vi "Set State_Measure SMU_HOLD.vi"(4 "Hold Time (s)":dbl=1.0 caption="Delay Time (s)", 6 "SMU Settings":T2={"Level"=0.01, "Level Range"=0.1, "Limit"=1.0, "Limit Range"=6.0, "Sense"=1009} {"Sense" items=["Local"=1008, "Remote"=1009]}, 7 "script name":string, 8 "error in (no error)":errorcluster, 9 "Published Data Id":string, 10 "Pins":string[](array[string])=["VDD"], 11 "Semiconductor Module Context":T3) -> (0 "error Out":errorcluster)   [LabVIEW 2013]
uses:
  <vilib>/NI_TestStand_SemiconductorModule/NI_TestStand_Semiconductor_Module.lvlibp/PinMap/General/SemiconductorModuleContext.ctl
  <instrlib>/niDCPower/nidcpower.llb/niDCPower Sense.ctl
  <instrlib>/niHSDIO/niHSDIO.llb/niHSDIO_ctl Trigger Script - trigID Values (Ring).ctl
  <vilib>/NI_TestStand_SemiconductorModule/NI_TestStand_Semiconductor_Module.lvlibp
panel:
  out "R Array":dbl[][](array[numeric]) format="%#_6p"
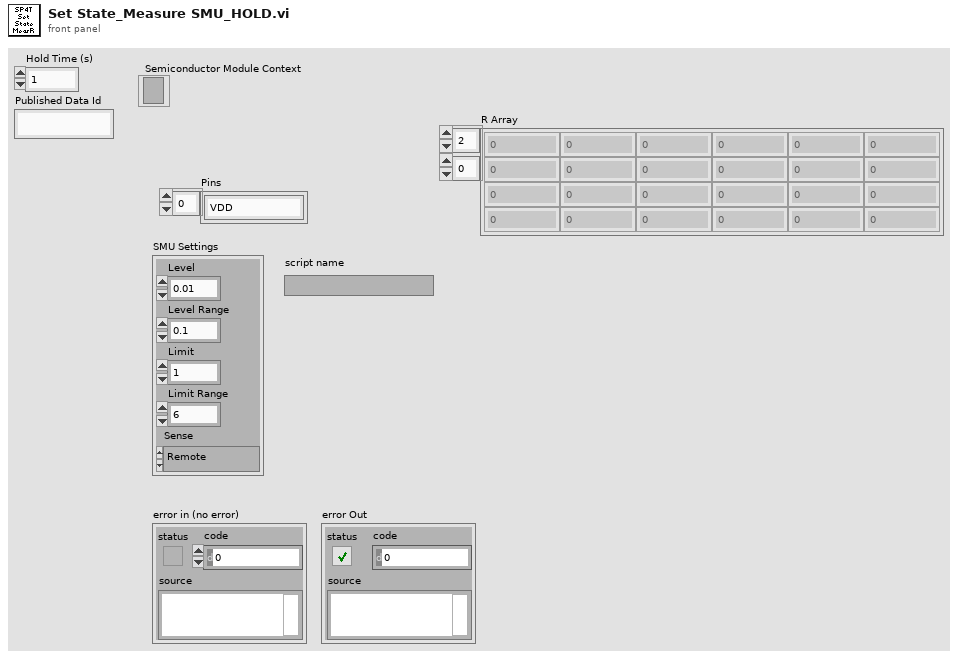
[diagram p1: front panel]
types:
  T1 = typedef "niDCPower Sense.ctl" = i32
  T2 = cluster{"Level":dbl, "Level Range":dbl, "Limit":dbl, "Limit Range":dbl, "Sense":T1}
  T3 = typedef "NI_TestStand_Semiconductor_Module.lvlibp/SemiconductorModuleContext.ctl" = refnum<k7>
  T4 = typedef "niHSDIO_ctl Trigger Script - trigID Values (Ring).ctl" = string
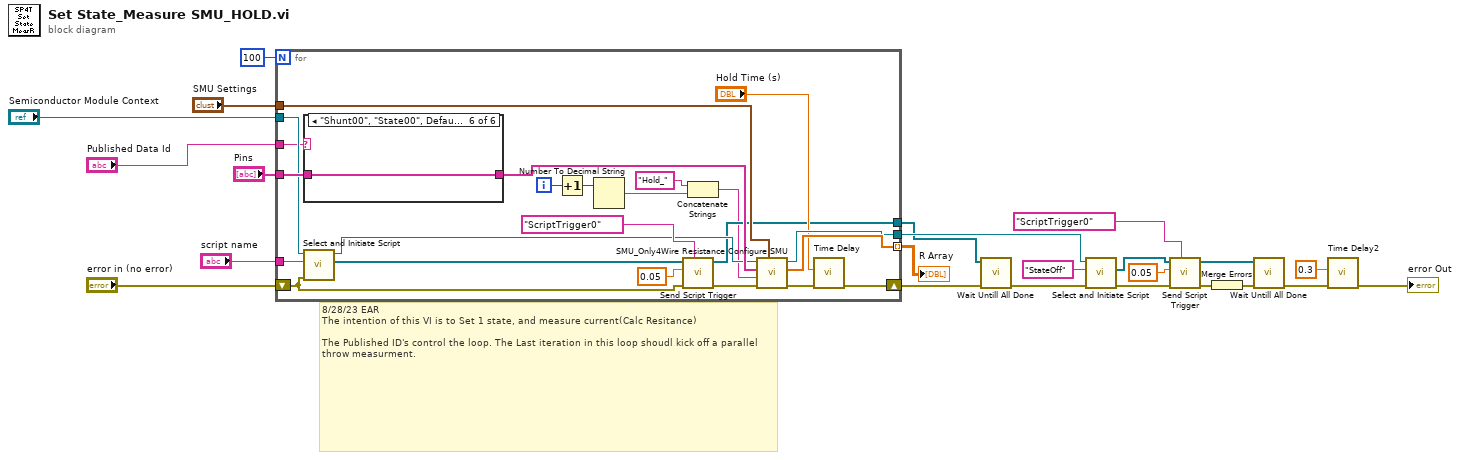
[diagram p0: block diagram]
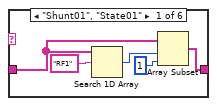
[diagram p2: hidden frame]
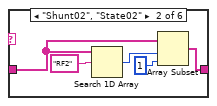
[diagram p3: hidden frame]
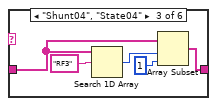
[diagram p4: hidden frame]
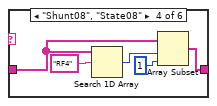
[diagram p5: hidden frame]
diagram:
  # "8/28/23 EAR\nThe intention of this VI is to Set 1 state, and measure current(Calc Resitance)\n\nThe Published ID's control the loop. The Last iteration in this loop shoudl kick off a parallel throw measurment."
  n1 = for {
    N: 100 -> [_]
    tunnel: "SMU Settings" -> [w46]
    tunnel: "Pins" -> [w42]
    tunnel: [w43] -> w21 mode=indexing
    shift-right: [w32] -> w6
    shift-left: "error in (no error)" -> [w35]
    tunnel: "Semiconductor Module Context" -> [w37]
    tunnel: "script name" -> [w36]
    tunnel: [w34] -> w11
    tunnel: "Published Data Id" -> [w30]
    tunnel: [w29] -> w4
    i -> [w25]
    n2 = case shown="\"Shunt00\", \"State00\", Default" w30 {
      tunnel: w42 -> [w50 w53 w60 w62 w67 w68]
      tunnel: [w49 w52 w59 w63 w67 w68] -> w41
      frame "Shunt01", "State01" {
        n3 = Search 1D Array(1D array=w50, element="RF1") -> (index of element=w48:i32)  [unwired: 1 in]
        n4 = Array Subset(array=w50, index=w48, length=1) -> (w49:string[])
      }
      frame "Shunt02", "State02" {
        n5 = Search 1D Array(1D array=w53, element="RF2") -> (index of element=w55:i32)  [unwired: 1 in]
        n6 = Array Subset(array=w53, index=w55, length=1) -> (w52:string[])
      }
      frame "Shunt04", "State04" {
        n7 = Search 1D Array(1D array=w60, element="RF3") -> (index of element=w58:i32)  [unwired: 1 in]
        n8 = Array Subset(array=w60, index=w58, length=1) -> (w59:string[])
      }
      frame "Shunt08", "State08" {
        n9 = Search 1D Array(1D array=w62, element="RF4") -> (index of element=w65:i32)  [unwired: 1 in]
        n10 = Array Subset(array=w62, index=w65, length=1) -> (w63:string[])
      }
      frame "Shunt15", "State15" {
      }
      frame "Shunt00", "State00", Default {
      }
    }
    n11 = call "Select and Initiate Script.vi"("error in (no error)"=w35, "script name"=w36, "Semiconductor Module Context"=w37) -> ("HSDIO GEN Sessions Out"=w39:refnum<k15>[], "Semiconductor Module Context Out"=w38:T3)  [unwired: 6 in, 1 out]
    n12 = Increment(x=w25) -> (x+1=w24:i32)
    n13 = Number To Decimal String(number=w24) -> (decimal integer string=w27:string)  [unwired: 1 in]
    n14 = call "Send Script Trigger.vi"("trigger id (script trigger 0)"=T4 "ScriptTrigger0", "error in (no error)"=w35, "Delay Time (s)"=0.05, "HSDIO Sessions In"=w39) -> ("error out"=w44:errorcluster, "HSDIO Sessions Out"=w29:refnum<k15>[])  [unwired: 6 in]
    n15 = Concatenate Strings("Hold_" ("string"), w27) -> (w26:string)
    n16 = call "SMU_Only4Wire Resistance Configure SMU.vi"("SMU Settings"=w46, "error in (no error)"=w44, "Published Data Id"=w26, "Pins"=w41, "Semiconductor Module Context"=w38) -> ("error Out"=w33:errorcluster, "R Array"=w43:dbl[], "Semiconductor Module Context Out"=w34:T3)  [unwired: 4 in]
    n17 = call "Time Delay"("error in (no error)"=w33, "Delay Time (s)"="Hold Time (s)") -> ("error out"=w32:errorcluster)  [unwired: 9 in]
  }
  "R Array" <- w21
  n18 = call "Wait Untill All Done.vi"("error in (no error)"=w6, "HSDIO Sessions In"=w4) -> ("error out"=w5:errorcluster)  [unwired: 8 in, 1 out]
  n19 = call "Select and Initiate Script.vi"("error in (no error)"=w5, "script name"="StateOff", "Semiconductor Module Context"=w11) -> ("error out"=w12:errorcluster, "HSDIO GEN Sessions Out"=w9:refnum<k15>[])  [unwired: 6 in, 1 out]
  n20 = call "Send Script Trigger.vi"("trigger id (script trigger 0)"=T4 "ScriptTrigger0", "error in (no error)"=w12, "Delay Time (s)"=0.05, "HSDIO Sessions In"=w9) -> ("error out"=w18:errorcluster, "HSDIO Sessions Out"=w17:refnum<k15>[])  [unwired: 6 in]
  n21 = Merge Errors(w18) -> (w20:errorcluster)
  n22 = call "Wait Untill All Done.vi"("error in (no error)"=w20, "HSDIO Sessions In"=w17) -> ("error out"=w3:errorcluster)  [unwired: 8 in, 1 out]
  n23 = call "Time Delay2"("error in (no error)"=w3, "Delay Time (s)"=0.3) -> ("error out"=→"error Out":errorcluster)  [unwired: 9 in]
